vi "Create Archiving Transaction List.vi"(9 "Combined LBCBs":bool, 10 "IsStep":T2, 11 "Number of LBCBs":T1) -> (2 "Transactions":T3[](array[typedef]))   [LabVIEW 2009]
uses:
  Dataset Transaction Id.ctl
  Dataset Source.ctl
  Dataset Type.ctl
  Apps/Yes No Button.ctl
  Data Access Objects/Application/Number Of LBCBs.ctl
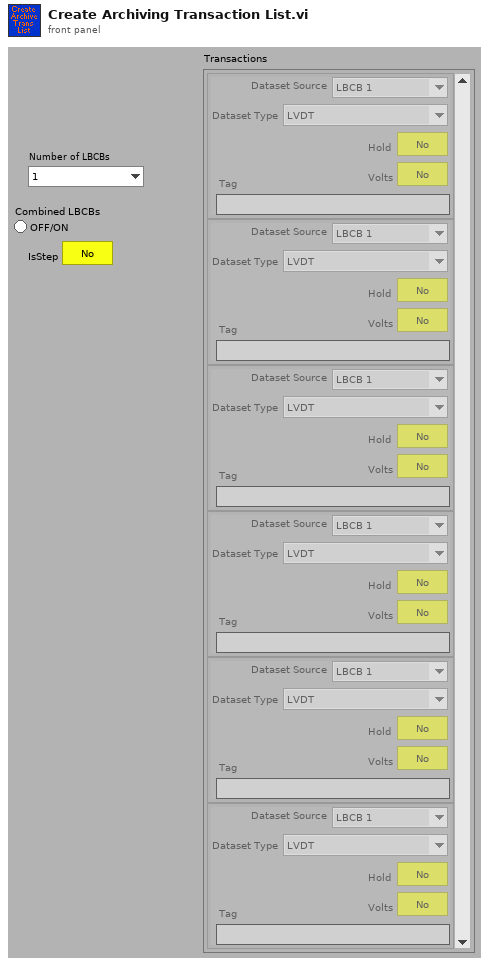
[diagram p1: front panel]
types:
  T1 = typedef "Number Of LBCBs.ctl" = enum16{"1", "2"}
  T2 = typedef "Yes No Button.ctl" = bool
  T3 = typedef "Dataset Transaction Id.ctl" = cluster{"Dataset Source":T4, "Dataset Type":T5, "Hold":T2, "Volts":T2, "Tag":string}
  T4 = typedef "Dataset Source.ctl" = enum16{"LBCB 1", "LBCB 2", "Combined", "External Sensors"}
  T5 = typedef "Dataset Type.ctl" = enum16{"LVDT", "Load Cell", "Actuator Command", "Servo Error", "Displacement Command", "Displacement", "Force"}
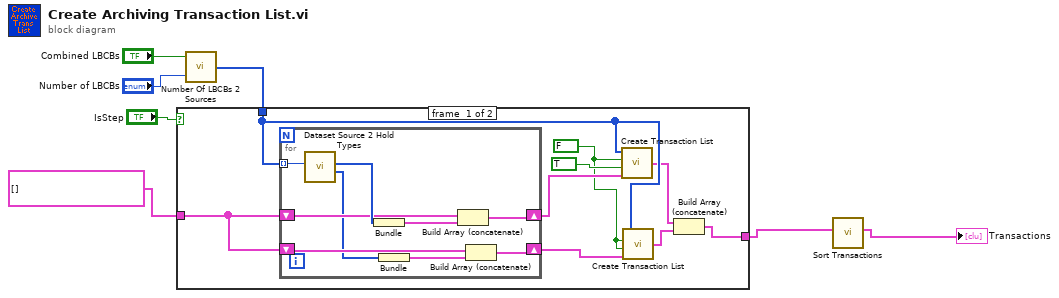
[diagram p0: block diagram]
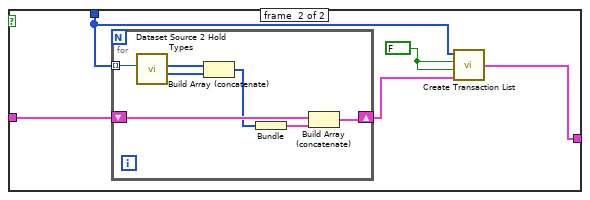
[diagram p2: hidden frame]
diagram:
  n1 = call "Number Of LBCBs 2 Sources.vi"("Number of LBCBs"="Number of LBCBs", "Combined LBCBs"="Combined LBCBs") -> ("Sources"=w4:T4[])
  n2 = case shown="False" "IsStep" {
    tunnel: w4 -> [w11 w28]
    tunnel: cluster{"Hold Types":T5[]}[] [] -> [w16 w30]
    tunnel: [w15 w27] -> w2
    frame #0 {
      w12 = FALSE ("Volts")
      n3 = for {
        tunnel: w11 -> [w25] mode=indexing
        shift-right: [w24] -> w14
        shift-left: w16 -> [w22]
        shift-right: [w19] -> w8
        shift-left: w16 -> [w18]
        n4 = call "Dataset Source 2 Hold Types.vi"("Dataset Source"=w25) -> ("No Holds Types Out"=w17:T5[], "Hold Types"=w23:T5[])  [unwired: 9 in]
        n5 = Bundle("Hold Types"=w23) -> (w21:cluster{"Hold Types":T5[]})  [unwired: 1 in]
        n6 = Bundle("No Holds Types Out"=w17) -> (w20:cluster{"No Holds Types Out":T5[]})  [unwired: 1 in]
        n7 = Build Array (concatenate)(w22, w21) -> (w24:cluster{"Hold Types":T5[]}[])
        n8 = Build Array (concatenate)(w18, w20) -> (w19:cluster{"No Holds Types Out":T5[]}[])
      }
      n9 = call "Create Transaction List.vi"("Source Types"=w14, "Hold"=T2 TRUE, "Volts"=w12, "Sources"=w11) -> ("Transactions"=w9:T3[])
      n10 = call "Create Transaction List.vi"("Source Types"=w8, "Hold"=w12, "Volts"=w12, "Sources"=w11) -> ("Transactions"=w10:T3[])
      n11 = Build Array (concatenate)(w9, w10) -> (w15:T3[])
    }
    frame #1 {
      w26 = FALSE ("Volts")
      n12 = for {
        tunnel: w28 -> [w37] mode=indexing
        shift-right: [w36] -> w29
        shift-left: w30 -> [w34]
        n13 = call "Dataset Source 2 Hold Types.vi"("Dataset Source"=w37) -> ("No Holds Types Out"=w31:T5[], "Hold Types"=w35:T5[])  [unwired: 9 in]
        n14 = Build Array (concatenate)(w35, w31) -> (w32:T5[])
        n15 = Bundle(w32) -> (w33:cluster{T5[]})  [unwired: 1 in]
        n16 = Build Array (concatenate)(w34, w33) -> (w36:cluster{"Hold Types":T5[]}[])
      }
      n17 = call "Create Transaction List.vi"("Source Types"=w29, "Hold"=w26, "Volts"=w26, "Sources"=w28) -> ("Transactions"=w27:T3[])
    }
  }
  n18 = call "Sort Transactions.vi"("Transactions In"=w2) -> ("Transactions Out"=→"Transactions":T3[])  [unwired: 10 in]
